vi "Tool_Unicode Update Tab Control Pages.vi"(5 "Interpret as Unicode (T)":bool=TRUE, 6 "error in":errorcluster, 7 "Page Captions":string[](array[string]), 9 "Tab Control":refnum<vi>) -> (0 "error out":errorcluster, 3 "Tab Control":refnum<vi>)   [LabVIEW 2009]
uses:
  _subVIs/tool_Unicode_Convert ASCII to Unicode (Scalar).vi
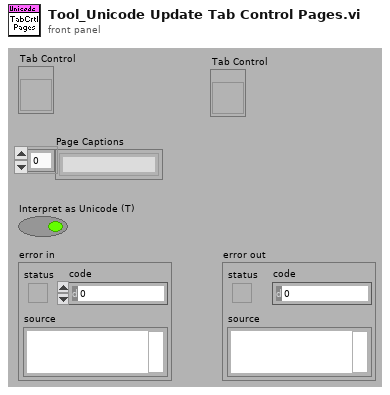
[diagram p1: front panel]
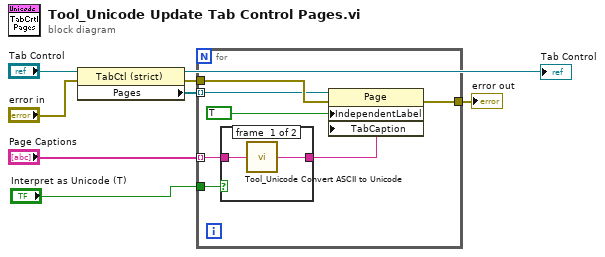
[diagram p0: block diagram]
diagram:
  n1 = property class="TabCtl (strict)"(reference="Tab Control", error in="error in") -> (reference out=→"Tab Control":refnum<vi>, error out=w6:errorcluster, "Pages"=w5:refnum<vi>[])
  n2 = for {
    tunnel: w5 -> [w14] mode=indexing
    tunnel: w6 -> [w15]
    tunnel: "Page Captions" -> [w10] mode=indexing
    tunnel: [w12] -> w8
    tunnel: "Interpret as Unicode (T)" -> [w11]
    n3 = case shown="False" w11 {
      tunnel: [w16 w18] -> w9
      tunnel: w10 -> [w17 w18]
      frame #0 {
        n4 = call-poly "Tool_Unicode Convert ASCII to Unicode.vi"("ASCII"=w17) -> ("Unicode"=w16:string)  [unwired: 4 in]
      }
      frame #1 {
      }
    }
    n5 = property class="Page"(reference=w14, error in=w15, "IndependentLabel"=TRUE ("Independent Label"), "TabCaption"=w9) -> (error out=w12:errorcluster)  [unwired: 1 out]
  }
  "error out" <- w8
